vi "OAT Polyphase Form.vi"(11 "filter":cluster{"coefficients":dbl[], "factor":i32} {"coefficients" format="%.2f"}) -> (1 "sub filter len":i32, 2 "decimate factor":i32, 3 "poly-phase filters":dbl[][](array[numeric]) format="%.2f")   [LabVIEW 2017, in "SoundVib_Resampling.lvlib"]
uses:
  <vilib>/addons/Sound and Vibration/Order Analysis/Resample Order Tracking/SoundVib_Resampling.lvlib
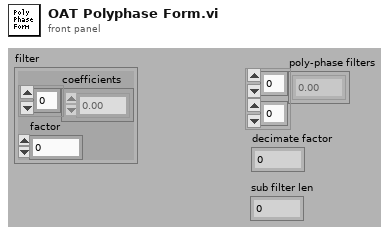
[diagram p1: front panel]
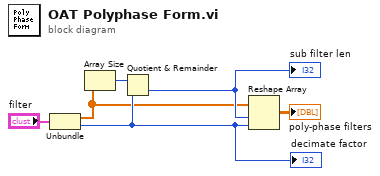
[diagram p0: block diagram]
diagram:
  n1 = Unbundle("filter") -> ("coefficients"=w1:dbl[], "factor"=w6:i32)
  "decimate factor" <- w6
  n2 = Array Size(array=w1) -> (size(s)=w4:i32)
  n3 = Quotient & Remainder(x=w4, y=w6) -> (floor(x/y)=w5:i32)  [unwired: 1 out]
  "sub filter len" <- w5
  n4 = Reshape Array(w1, w5, w6) -> (→"poly-phase filters":dbl[][])
